vi "Close.vi"(8 "error in (no error)":errorcluster, 11 "Tektronix MSO5 in":refnum<class "Tektronix MSO5.lvclass">) -> (0 "error out":errorcluster, 3 "Tektronix MSO5 out":refnum<class "Tektronix MSO5.lvclass">)   [LabVIEW 2025, in "Scope.lvlib" / "Tektronix MSO5.lvclass"]
uses:
  Tektronix MSO5.lvclass
  Tektronix MSO5.lvclass/Tektronix MSO5.ctl
  <instrlib>/Tektronix MSO5 Series/Utilities/MS058LP Library.lvlib
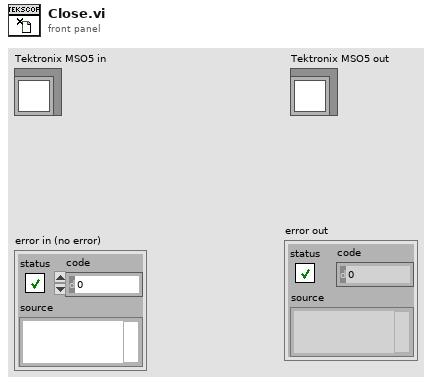
[diagram p1: front panel]
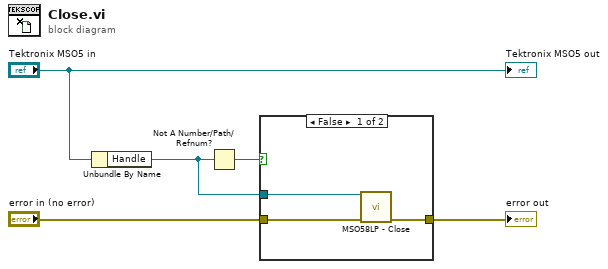
[diagram p0: block diagram]
diagram:
  n1 = Unbundle By Name("Tektronix MSO5 in") -> ("Handle"=w2:refnum<visa-resource-name>)
  n2 = Not A Number/Path/Refnum?(number/path/refnum=w2) -> (NaN/Path/Refnum?=w1:bool)
  n3 = case shown="False" w1 {
    tunnel: [w7 w9] -> w5
    tunnel: "error in (no error)" -> [w8 w9]
    tunnel: w2 -> [w6 _]
    frame False {
      n4 = call <instrlib>:"MSO58LP - Close.vi"("error in"=w8, "VISA In"=w6) -> ("error out"=w7:errorcluster)  [unwired: 9 in]
    }
    frame True {
    }
  }
  "error out" <- w5
  "Tektronix MSO5 out" <- "Tektronix MSO5 in"
